vi "XB Hear.vi"(0 "VISA resource name":refnum<visa-resource-name>, 1 "error in (no error)":errorcluster) -> (2 "VISA resource name out":refnum<visa-resource-name>, 3 "String Received":string, 4 "error out":errorcluster)   [LabVIEW 2014]
doc: "The VI reads the return string from a XB PC SEND operation. A \"\\n\" LF is expected to terminate the string. If the time is exceeded or if more than 127 characters are received an error is generated."
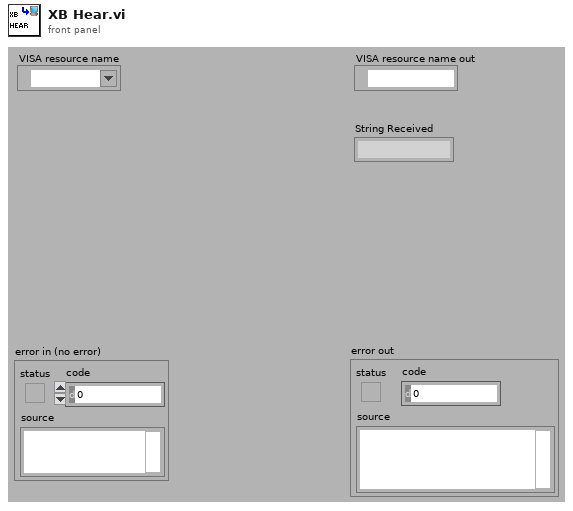
[diagram p1: front panel]
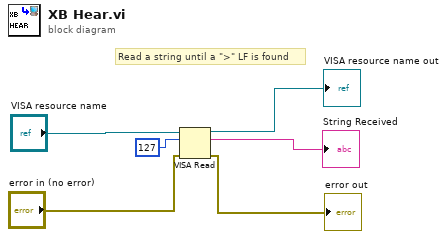
[diagram p0: block diagram]
diagram:
  # "Read a string until a \">\" LF is found"
  n1 = VISA Read(VISA resource name="VISA resource name", byte count=u32 127, error in (no error)="error in (no error)") -> (VISA resource name out=→"VISA resource name out":refnum<visa-resource-name>, read buffer=→"String Received":string, error out=→"error out":errorcluster)  [unwired: 1 out]
